vi "Multistate LED Example LV2016 NIVerified.vi"() -> ()   [LabVIEW 2016]
panel:
  in  "stop":bool
  out "Color Box":u32(colorbox)
  in  "Enum":T1(ring)
  # "Overview:\nThis example uses a customized color box control to represent a multicolor LED\nRequirements:\nLabVIEW 2012 (or compatible).\nInstructions:\nSince the color box control is actually a U32 numeric, you can wire in any value from 0 to 4,294,967,295, however, the easiest way is usually to use a color box constant on the block diagram to assign a value to the multi-state LED indicator. Using this in conjunction with a Case Structure and then some sort of selection control, such as an enum, provides an easy way to use this multi-state LED indicator."
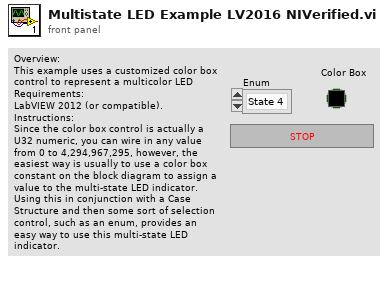
[diagram p1: front panel]
types:
  T1 = enum16{"State 4", "State 3", "State 2", "State 1", "State 0"}
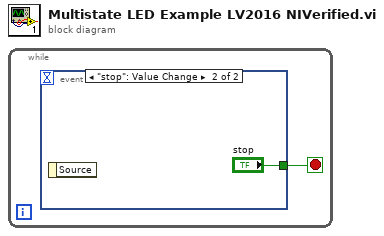
[diagram p0: block diagram]
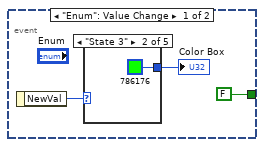
[diagram p2: hidden frame]
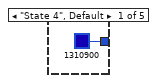
[diagram p3: hidden frame]
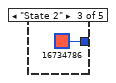
[diagram p4: hidden frame]
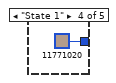
[diagram p5: hidden frame]
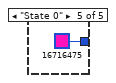
[diagram p6: hidden frame]
diagram:
  n1 = while {
    stop <- w1 stop-if-true
    n2 = event shown="[1] \"stop\": Value Change" {
      selector: _ -> [_ _]
      dyn-events: _ -> [_ _]
      timeout: _ -> [_ _]
      tunnel: [FALSE ("stop") "stop"] -> w1
      event "Enum": Value Change {
        n3 = event-data() -> ("NewVal"=w3:T1)  [unwired: 1 in]
        n4 = case shown="\"State 3\"" w3 {
          tunnel: [u32 1310900 u32 786176 u32 16734786 u32 11771020 u32 16716475] -> w4
          frame "State 4", Default {
          }
          frame "State 3" {
          }
          frame "State 2" {
          }
          frame "State 1" {
          }
          frame "State 0" {
          }
        }
        "Color Box" <- w4
      }
      event "stop": Value Change {
        n5 = event-data() -> ()  [unwired: 1 in, 1 out]
      }
    }
  }
